vi "Read All Param.vi"(8 "error in (no error)":errorcluster, 11 "Data1D in":refnum<class "Data1D.lvclass">) -> (0 "error out":errorcluster, 1 "dt":dbl, 2 "1D Array":dbl[](array[numeric]), 3 "Data1D out":refnum<class "Data1D.lvclass">, 4 "t0":dbl)   [LabVIEW 2014, in "Data1D.lvclass"]
uses:
  Data1D.lvclass
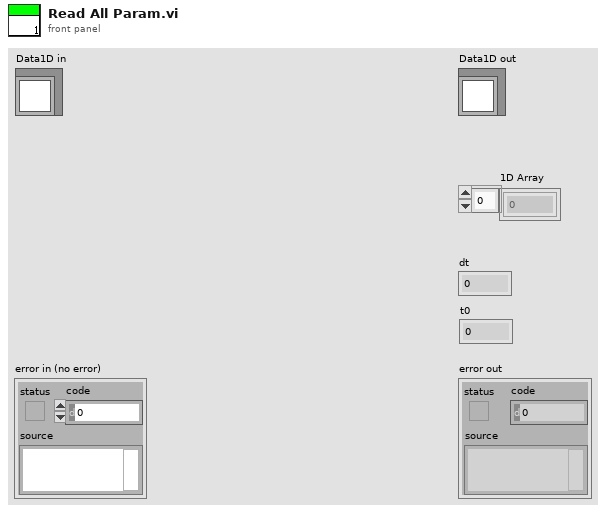
[diagram p1: front panel]
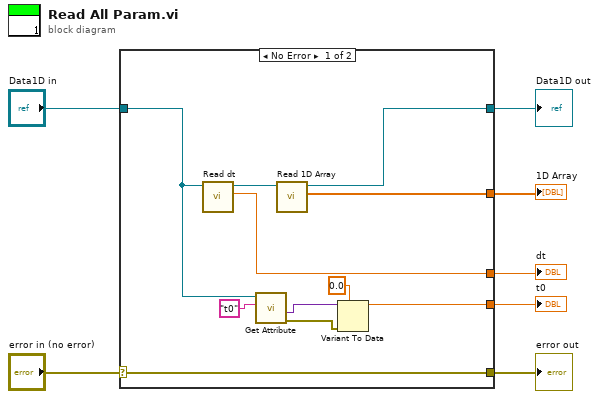
[diagram p0: block diagram]
diagram:
  n1 = case shown="No Error" "error in (no error)" {
    selector: "error in (no error)" -> [w14 w20]
    tunnel: [w14 w20] -> w6
    tunnel: [w17 w19] -> w4
    tunnel: "Data1D in" -> [w9 w19]
    tunnel: [w15 _] -> w3
    tunnel: [w16 _] -> w2
    tunnel: [w8 _] -> w1
    frame No Error {
      n2 = call "Read dt.vi"("Data1D in"=w9) -> ("dt"=w16:dbl, "Data1D out"=w18:refnum<class "Data1D.lvclass">)  [unwired: 8 in, 1 out]
      n3 = call-dynamic "Get Attribute.vi"("Name"="t0", "AbstractData in"=w9) -> ("error out"=w12:errorcluster, "value"=w11:variant)  [unwired: 6 in, 2 out]
      n4 = call "Read 1D Array.vi"("Data1D in"=w18) -> ("1D Array"=w15:dbl[], "Data1D out"=w17:refnum<class "Data1D.lvclass">)  [unwired: 8 in, 1 out]
      n5 = Variant To Data(error in=w12, type=0.0, Variant=w11) -> (data=w8:dbl)  [unwired: 1 out]
    }
    frame Error {
    }
  }
  "error out" <- w6
  "Data1D out" <- w4
  "1D Array" <- w3
  "dt" <- w2
  "t0" <- w1
